vi "Execute Test - Template Method.vi"   [LabVIEW 2020, in "Test.lvclass"]
uses:
  Test.lvclass
  XML Report/XML Report.lvclass
  JSON Report/JSON Report.lvclass
  Web Reports/Web Reports.lvclass
  Slideshow Report/Slideshow Report.lvclass
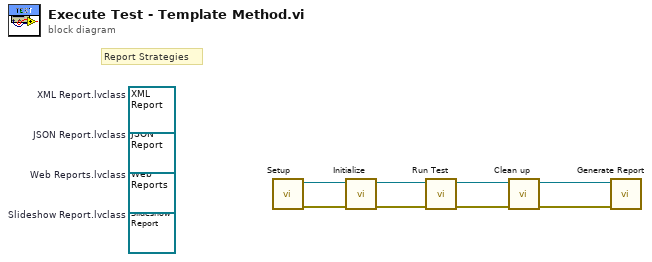
[diagram p0: block diagram]
diagram:
  (unwired) refnum<class "Slideshow Report.lvclass"> refnum  # Slideshow Report.lvclass
  (unwired) refnum<class "Web Reports.lvclass"> refnum  # Web Reports.lvclass
  (unwired) refnum<class "JSON Report.lvclass"> refnum  # JSON Report.lvclass
  (unwired) refnum<class "XML Report.lvclass"> refnum  # XML Report.lvclass
  # "Report Strategies"
  n1 = call "Setup.vi"() -> ("error out"=w7:errorcluster, "Test out"=w8:refnum<class "Test.lvclass">)  [unwired: 10 in]
  n2 = call "Initialize.vi"("error in (no error)"=w7, "Test in"=w8) -> ("error out"=w5:errorcluster, "Test out"=w6:refnum<class "Test.lvclass">)  [unwired: 8 in]
  n3 = call "Run Test.vi"("error in (no error)"=w5, "Test in"=w6) -> ("error out"=w3:errorcluster, "Test out"=w4:refnum<class "Test.lvclass">)  [unwired: 8 in]
  n4 = call "Clean up.vi"("error in (no error)"=w3, "Test in"=w4) -> ("error out"=w1:errorcluster, "Test out"=w2:refnum<class "Test.lvclass">)  [unwired: 8 in]
  n5 = call "Generate Report.vi"("error in (no error)"=w1, "Test in"=w2) -> ()  [unwired: 8 in, 2 out]
